vi "InsertCoin.vi"(8 "error in (no error)":errorcluster, 11 "NoCoinState in":refnum<class "NoCoinState.lvclass">) -> (0 "error out":errorcluster, 1 "NextState":T1=enum."有硬幣", 2 "ProcessMessage":string, 3 "NoCoinState out":refnum<class "NoCoinState.lvclass">)   [LabVIEW 2013, in "NoCoinState.lvclass"]
uses:
  NoCoinState.lvclass
  StateMark.ctl
panel:
  # "投入硬幣動作"
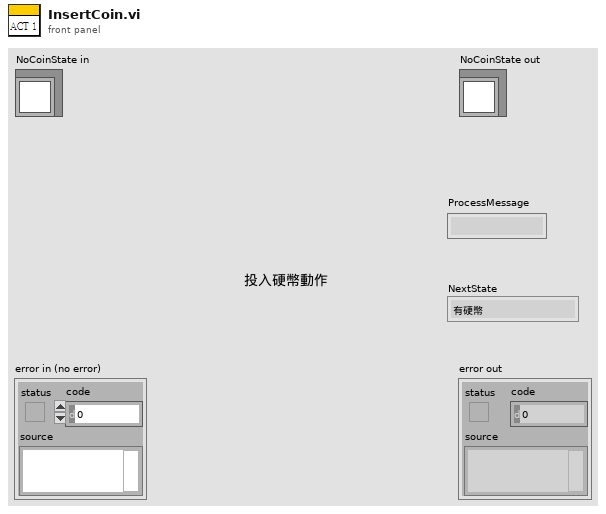
[diagram p1: front panel]
types:
  T1 = typedef "StateMark.ctl" = enum16{"沒有硬幣", "有硬幣", "賣出糖果", "糖果賣完", "NoChange"}
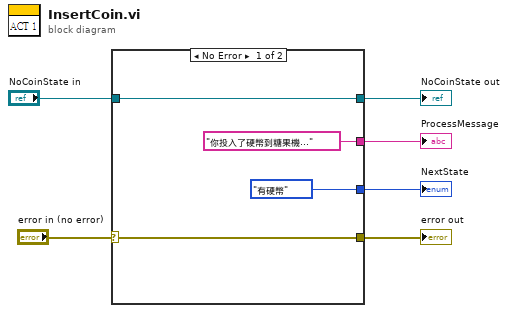
[diagram p0: block diagram]
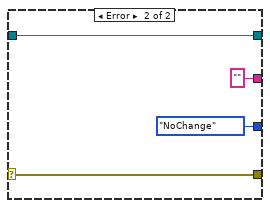
[diagram p2: hidden frame]
diagram:
  n1 = case shown="No Error" "error in (no error)" {
    selector: "error in (no error)" -> [w9 w13]
    tunnel: [w10 w14] -> w5
    tunnel: "NoCoinState in" -> [w10 w14]
    tunnel: [w9 w13] -> w3
    tunnel: ["你投入了硬幣到糖果機..." ("ProcessMessage") "" ("ProcessMessage")] -> w2
    tunnel: [StateMark."有硬幣" ("NextState") StateMark."NoChange" ("NextState")] -> w1
    frame No Error {
    }
    frame Error {
    }
  }
  "error out" <- w3
  "NoCoinState out" <- w5
  "NextState" <- w1
  "ProcessMessage" <- w2
